vi "Serial_port.vi"() -> ()   [LabVIEW 2013]
uses:
  <vilib>/Instr/_visa.llb/VISA Configure Serial Port (Instr).vi
panel:
  in  "Absloute  2":bool
  in  "Absloute":bool
  in  "Set orign":bool
  in  "single mode command":string
  in  "start single mode":bool
  out "error out 3":errorcluster
  out "read buffer":string
  out "error out 2":errorcluster
  in  "stop":bool
  in  "baud rate (9600) 2":u32=9600
  in  "VISA resource name 2":refnum<visa-resource-name>
  in  "VISA resource name":refnum<visa-resource-name>
  in  "baud rate (9600)":u32=9600
  # "Read Terminal"
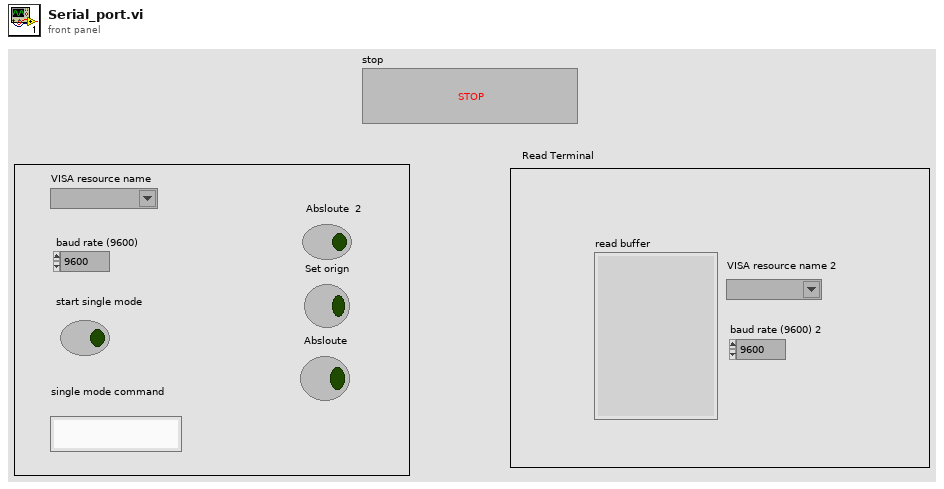
[diagram p1: front panel]
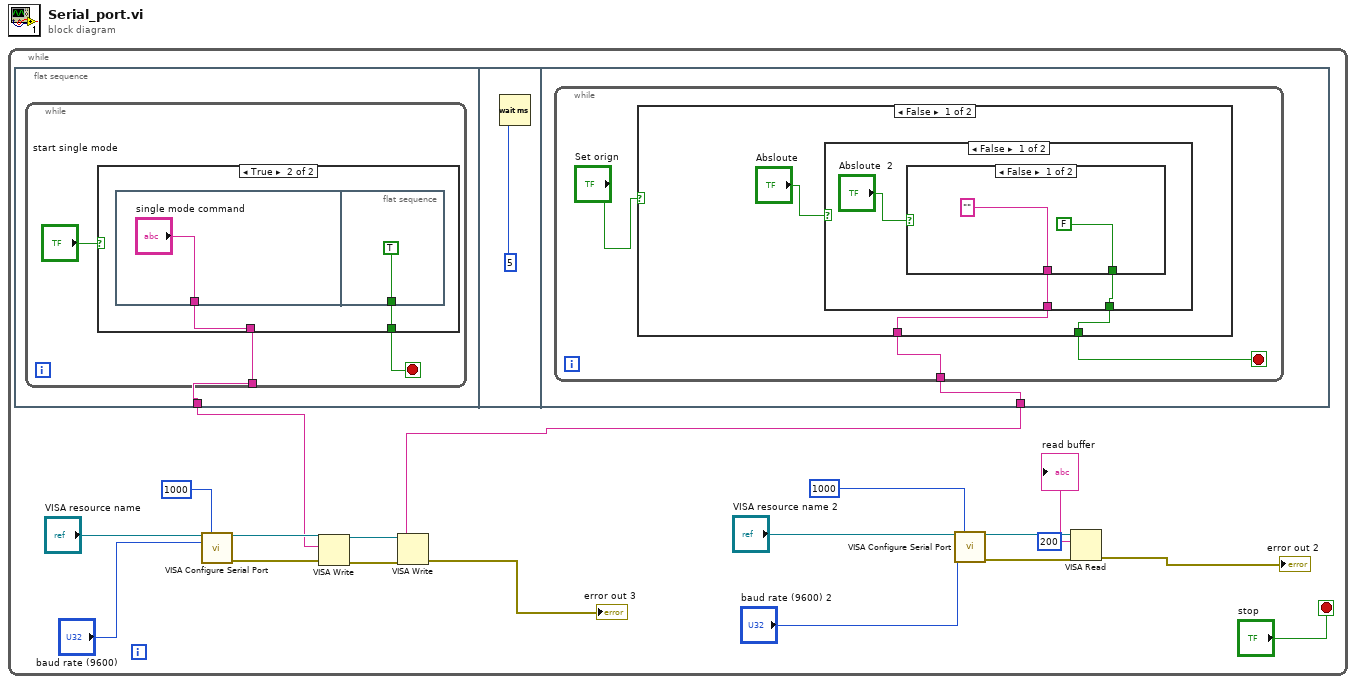
[diagram p0: block diagram]
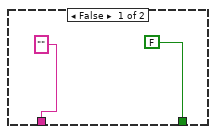
[diagram p2: hidden frame]
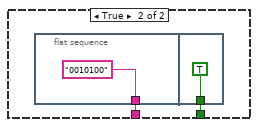
[diagram p3: hidden frame]
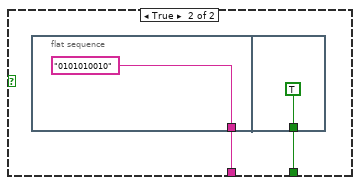
[diagram p4: hidden frame]
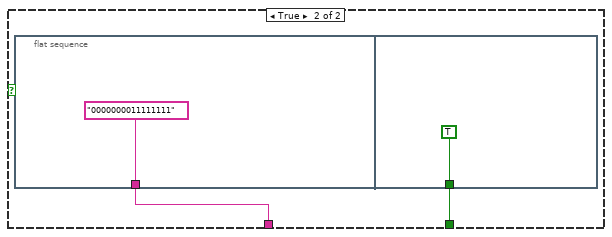
[diagram p5: hidden frame]
diagram:
  n1 = while {
    stop <- "stop" stop-if-true
    n2 = flat-sequence {
      tunnel: [w20] -> w2
      tunnel: [w31] -> w1
      frame #0 {
        n3 = while {
          tunnel: [w22] -> w20
          stop <- w21 stop-if-true
          n4 = case shown="True" "start single mode" {
            tunnel: ["" w27] -> w22
            tunnel: [FALSE w26] -> w21
            frame False {
            }
            frame True {
              n5 = flat-sequence {
                tunnel: ["single mode command"] -> w27
                tunnel: [TRUE] -> w26
                frame #0 {
                }
                frame #1 {
                }
              }
            }
          }
        }
      }
      frame #1 {
        n6 = Wait (ms)(milliseconds to wait=u32 5) -> ()  [unwired: 1 out]
      }
      frame #2 {
        n7 = while {
          tunnel: [w33] -> w31
          stop <- w32 stop-if-true
          n8 = case shown="False" "Set orign" {
            tunnel: [w37 w52] -> w33
            tunnel: [w35 w51] -> w32
            frame False {
              n9 = case shown="False" "Absloute" {
                tunnel: [w40 w48] -> w37
                tunnel: [w38 w47] -> w35
                frame False {
                  n10 = case shown="False" "Absloute  2" {
                    tunnel: ["" w44] -> w40
                    tunnel: [FALSE w43] -> w38
                    frame False {
                    }
                    frame True {
                      n11 = flat-sequence {
                        tunnel: ["0010100"] -> w44
                        tunnel: [TRUE] -> w43
                        frame #0 {
                        }
                        frame #1 {
                        }
                      }
                    }
                  }
                }
                frame True {
                  n12 = flat-sequence {
                    tunnel: ["0101010010"] -> w48
                    tunnel: [TRUE] -> w47
                    frame #0 {
                    }
                    frame #1 {
                    }
                  }
                }
              }
            }
            frame True {
              n13 = flat-sequence {
                tunnel: ["0000000011111111"] -> w52
                tunnel: [TRUE] -> w51
                frame #0 {
                }
                frame #1 {
                }
              }
            }
          }
        }
      }
    }
    n14 = call-poly "VISA Configure Serial Port"("VISA resource name"="VISA resource name", "timeout (10sec)"=u32 1000, "baud rate (9600)"="baud rate (9600)") -> ("VISA resource name out"=w19:refnum<visa-resource-name>, "error out"=w18:errorcluster)  [unwired: 11 in]
    n15 = VISA Write(VISA resource name=w19, write buffer=w2, error in (no error)=w18) -> (VISA resource name out=w6:refnum<visa-resource-name>, error out=w5:errorcluster)  [unwired: 1 out]
    n16 = VISA Write(VISA resource name=w6, write buffer=w1, error in (no error)=w5) -> (error out=→"error out 3":errorcluster)  [unwired: 2 out]
    n17 = call-poly "VISA Configure Serial Port"("VISA resource name"="VISA resource name 2", "timeout (10sec)"=u32 1000, "baud rate (9600)"="baud rate (9600) 2") -> ("VISA resource name out"=w15:refnum<visa-resource-name>, "error out"=w14:errorcluster)  [unwired: 11 in]
    n18 = VISA Read(VISA resource name=w15, byte count=u32 200, error in (no error)=w14) -> (read buffer=→"read buffer":string, error out=→"error out 2":errorcluster)  [unwired: 2 out]
  }
